vi "_Read Spectrum.vi"(0 "file path":path, 3 "AcqMethod":T1[](array[typedef]) {"ScanType" format="%#.6g"; "Mass Range"."Res" items=["High/High", "Medium/Medium", "Low/Low", "High/Medium", "High/Low", "Medium/High", "Medium/Low", "Low/High", "Low/Medium"]}, 5 "Scan# (1-based)":i32=1, 7 "Expt# (1-based)":i32=1, 9 "MR# (1-based)":i32=1, 11 "error in (no error)":errorcluster) -> (1 "Expt# Out":i32=1, 2 "MR# Out":i32=1, 4 "Data":T6, 6 "Scan# out":i32=1, 10 "Version":i32, 12 "raw data":i32[](array[numeric]), 14 "XY Graph":cluster{dbl[], u32[]}(graph), 15 "error out":errorcluster)   [LabVIEW 2015]
uses:
  Type/_Data.ctl
  Type/_XML Expt.ctl
  Type/_XML Lens.ctl
  Type/_Mass Range Property.ctl
  Type/_Mass Range Parameters.ctl
  Type/_RT Res Type.ctl
panel:
  out "Index Array":i64[][](array[numeric])
  out "Steps":i32[][](array[numeric])
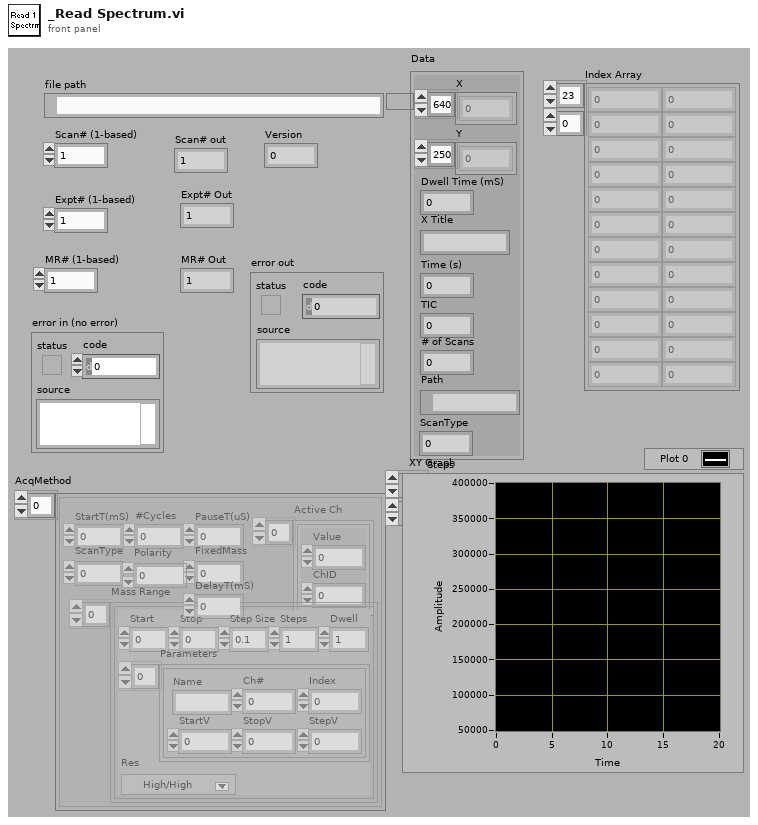
[diagram p1: front panel]
types:
  T1 = typedef "_XML Expt.ctl" = cluster{"StartT(mS)":i32, "#Cycles":i32, "PauseT(uS)":i32, "ScanType":i32, "Polarity":u8, "FixedMass":dbl, "DelayT(mS)":i32, "Active Ch":T2[], "Mass Range":T3[]}
  T2 = typedef "_XML Lens.ctl" = cluster{"Value":dbl, "ChID":u8}
  T3 = typedef "_Mass Range Property.ctl" = cluster{"Start":dbl, "Stop":dbl, "Step Size":dbl, "Steps":i32, "Dwell":dbl, "Parameters":T4[], "Res":T5}
  T4 = typedef "_Mass Range Parameters.ctl" = cluster{"Name":string, "Ch#":u8, "StartV":dbl, "StopV":dbl, "StepV":dbl, "Index":u8}
  T5 = typedef "_RT Res Type.ctl" = u16
  T6 = typedef "_Data.ctl" = cluster{"X":dbl[], "Y":dbl[], "Dwell Time (mS)":dbl, "X Title":string, "Time (s)":dbl, "TIC":u32, "# of Scans":i32, "Path":path, "ScanType":i32}
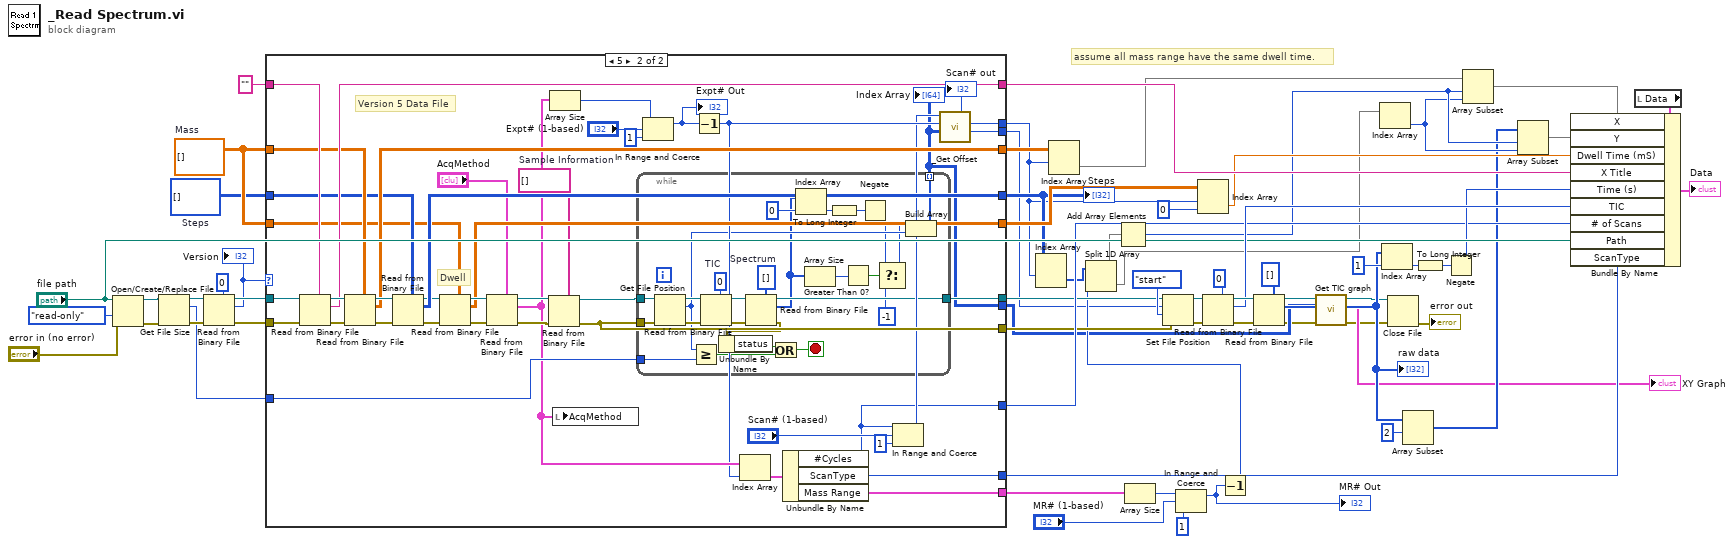
[diagram p0: block diagram]
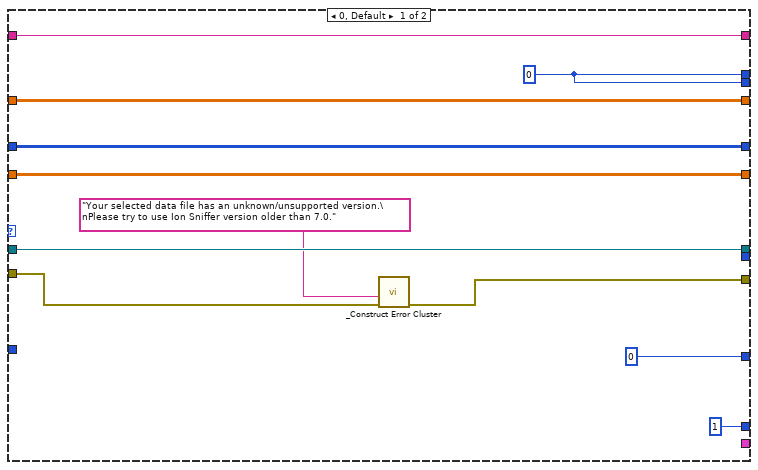
[diagram p2: hidden frame]
diagram:
  w31 = i32[][] []  # Steps
  w32 = dbl[][] []  # Mass
  # "assume all mass range have the same dwell time."
  n1 = Open/Create/Replace File(file path (use dialog)="file path", error in="error in (no error)", access (0:read/write)=enum16{"read/write", "read-only", "write-only"}."read-only") -> (refnum out=w56:refnum<file>, error out=w55:errorcluster)  [unwired: 4 out]
  n2 = Get File Size ("EOF")(file=w56, error in=w55) -> (refnum out=w44:refnum<file>, size (in bytes)=w40:i64, 0:w43:errorcluster)
  n3 = Read from Binary File(5:0 ("pos offset (0)"), 8:w43, 11:w44) -> (0:w41:errorcluster, 2:w29:i32, 3:w42:refnum<file>)  [unwired: 4 out]
  "Version" <- w29
  n4 = case shown="5" w29 {
    tunnel: w41 -> [w75 w116]
    tunnel: w42 -> [w76 w115]
    tunnel: [w70 w112] -> w33
    tunnel: [w71 w110] -> w37
    tunnel: [0 w78] -> w39
    tunnel: [w76 w100] -> w28
    tunnel: [w73 w96] -> w27
    tunnel: w40 -> [_ w99]
    tunnel: [w68 w111] -> w19
    tunnel: "" -> [w71 w109]
    tunnel: w32 -> [w70 w108]
    tunnel: w31 -> [w68 w107]
    tunnel: w32 -> [w69 w102]
    tunnel: [w69 w101] -> w35
    tunnel: [w66 w82] -> w18
    tunnel: [1 ("ScanType") w88] -> w24
    tunnel: [_ w86] -> w23
    tunnel: [w66 w80] -> w8
    tunnel: [_ w77] -> w6
    frame 0, Default {
      w66 = 0 ("lower limit")
      n5 = call "_Construct Error Cluster.vi"("error in"=w75, "reason"="Your selected data file has an unknown/unsupported version.\nPlease try to use Ion Sniffer version older than 7.0.") -> ("error out"=w73:errorcluster)  [unwired: 2 in, 3 out]
    }
    frame 5 {
      w94 = string[] []  # Sample Information
      # "Dwell"
      # "Version 5 Data File"
      n6 = Read from Binary File(5:w109, 8:w116, 11:w115) -> (0:w118:errorcluster, 2:w110:string, 3:w114:refnum<file>)  [unwired: 4 out]
      n7 = Read from Binary File(5:w108, 8:w118, 11:w114) -> (0:w117:errorcluster, 2:w112:dbl[][], 3:w113:refnum<file>)  [unwired: 4 out]
      n8 = Read from Binary File(5:w107, 8:w117, 11:w113) -> (0:w104:errorcluster, 2:w111:i32[][], 3:w105:refnum<file>)  [unwired: 4 out]
      n9 = Read from Binary File(5:w102, 8:w104, 11:w105) -> (0:w106:errorcluster, 2:w101:dbl[][], 3:w103:refnum<file>)  [unwired: 4 out]
      n10 = Read from Binary File(5:"AcqMethod", 8:w106, 11:w103) -> (0:w95:errorcluster, 2:w87:T1[], 3:w98:refnum<file>)  [unwired: 4 out]
      n11 = Read from Binary File(5:w94, 8:w95, 11:w98) -> (0:w96:errorcluster, 3:w97:refnum<file>)  [unwired: 5 out]
      n12 = Array Size(array=w87) -> (size(s)=w90:i32)
      n13 = local write "AcqMethod"(w87) -> ()
      n14 = while {
        tunnel: w97 -> [w143]
        tunnel: w96 -> [w142]
        tunnel: [w140] -> w100
        tunnel: w99 -> [w139]
        tunnel: [w125] -> w77 mode=indexing
        stop <- w136 stop-if-true
        w131 = u32 0  # TIC
        w141 = u32[] []  # Spectrum
        n15 = Get File Position(4:w142, 7:w143) -> (0:w132:errorcluster, 2:w126:i64, 3:w134:refnum<file>)
        n16 = Greater Or Equal?(x=w126, y=w139) -> (x >= y?=w137:bool)
        n17 = Read from Binary File(5:w131, 8:w132, 11:w134) -> (0:w135:errorcluster, 3:w133:refnum<file>)  [unwired: 5 out]
        n18 = Read from Binary File(5:w141, 8:w135, 11:w133) -> (0:w130:errorcluster, 2:w124:u32[], 3:w140:refnum<file>)  [unwired: 4 out]
        n19 = Unbundle By Name(w130) -> ("status"=w138:bool)
        n20 = Or(x=w138, y=w137) -> (x .or. y?=w136:bool)
        n21 = Index Array(array=w124, index=0) -> (element=w128:u32)
        n22 = Array Size(array=w124) -> (size(s)=w123:i32)
        n23 = To Long Integer(number=w128) -> (32bit integer=w129:i32)
        n24 = Greater Than 0?(x=w123) -> (x > 0?=w122:bool)
        n25 = Negate(x=w129) -> (-x=w121:i32)
        n26 = Select(t=w121, s=w122, f=-1) -> (s? t:f=w119:i32)
        n27 = Build Array(w119, w126) -> (w125:i64[])
      }
      "Index Array" <- w77
      n28 = In Range and Coerce(upper limit=w90, x="Expt# (1-based)", lower limit=1) -> (coerced(x)=w85:i32)  [unwired: 1 out]
      "Expt# Out" <- w85
      n29 = Decrement(x=w85) -> (x-1=w82:i32)
      n30 = Index Array(array=w87, index=w82) -> (element=w89:T1)
      n31 = Unbundle By Name(w89) -> ("#Cycles"=w78:i32, "ScanType"=w88:i32, "Mass Range"=w86:T3[])
      n32 = In Range and Coerce(upper limit=w78, x="Scan# (1-based)", lower limit=1) -> (coerced(x)=w81:i32)  [unwired: 1 out]
      n33 = call "_Get Offset.vi"("Index Array"=w77, "Expt# (0-based)"=w82, "Scan# (1-based)"=w81) -> ("Offset"=w80:i64, "Scan# out"=→"Scan# out":i32)  [unwired: 3 out]
    }
  }
  "Steps" <- w19
  n34 = Index Array(array=w19, index (row)=w18) -> (element=w17:i32[])  [unwired: 1 in]
  n35 = Index Array(array=w33, index (row)=w18) -> (element=w26:dbl[])  [unwired: 1 in]
  n36 = Array Size(array=w23) -> (size(s)=w21:i32)
  n37 = Set File Position(offset (in bytes) (0)=w8, refnum=w28, from (0:start)=enum16{"start", "end", "current"}."start" ("pos mode (0:2)"), error in=w27) -> (refnum out=w53:refnum<file>, error out=w52:errorcluster)
  n38 = In Range and Coerce(upper limit=w21, x="MR# (1-based)", lower limit=1) -> (coerced(x)=w16:i32)  [unwired: 1 out]
  "MR# Out" <- w16
  n39 = Index Array(array=w35, index (row)=w18, index (col)=0 ("index (row)")) -> (element=w34:dbl)
  n40 = Read from Binary File(5:u32 0, 8:w52, 11:w53) -> (0:w62:errorcluster, 2:w59:u32, 3:w63:refnum<file>)  [unwired: 4 out]
  n41 = Decrement(x=w16) -> (x-1=w15:i32)
  n42 = Split 1D Array(array=w17, index=w15) -> (first subarray=w14:i32[], second subarray=w13:i32[])
  n43 = Add Array Elements(numeric array=w14) -> (sum=w12:i32)
  n44 = Read from Binary File(5:u32[] [] ("Spectrum"), 8:w62, 11:w63) -> (0:w2:errorcluster, 2:w7:u32[], 3:w5:refnum<file>)  [unwired: 4 out]
  "raw data" <- w7
  n45 = call "Get TIC graph.vi"("error in"=w2, "Array"=w6, "Byte Stream File in"=w5) -> ("error out"=w1:errorcluster, "Cluster"=→"XY Graph":cluster{dbl[], u32[]}, "Byte Stream File out"=w4:refnum<file>)  [unwired: 6 in]
  n46 = Index Array(array=w13) -> (element=w11:i32)  [unwired: 1 in]
  n47 = Index Array(array=w7, index=1) -> (element=w50:u32)
  n48 = Close File(refnum=w4, error in=w1) -> (error out=→"error out":errorcluster)  [unwired: 1 out]
  n49 = Array Subset(array=w7, index=2) -> (w9:u32[])  [unwired: 1 in]
  n50 = To Long Integer(number=w50) -> (32bit integer=w48:i32)
  n51 = Negate(x=w48) -> (-x=w47:i32)
  n52 = Array Subset(array=w26, index=w12, length=w11) -> (w25:dbl[])
  n53 = Array Subset(array=w9, index=w12, length=w11) -> (w10:u32[])
  n54 = local read "Data"() -> (w60:T6)
  n55 = Bundle By Name(cluster=w60, "X"=w25, "Y"=w10, "Dwell Time (mS)"=w34, "X Title"=w37, "Time (s)"=w47, "TIC"=w59, "# of Scans"=w39, "Path"="file path", "ScanType"=w24) -> (→"Data":T6)
